vi "save_TIFF_U16array.vi"(8 "time_stamp":bool=TRUE, 9 "filename":string, 10 "Path":path=path "D:/datanew/seal/20160708_test", 11 "Image Pixels (U16)":u16[][](array[numeric])) -> ()   [LabVIEW 2014]
panel:
  out "error out":errorcluster
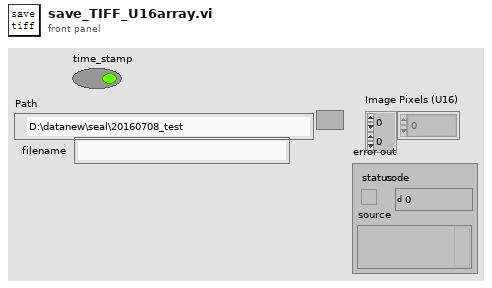
[diagram p1: front panel]
types:
  T1 = typedef "Image Type" = u32
  T2 = cluster{"Rows Per Strip":i32, "Photometric":i32, "Compression Type":i32}
  T3 = typedef "IMAQ Image.ctl" = refnum<image>
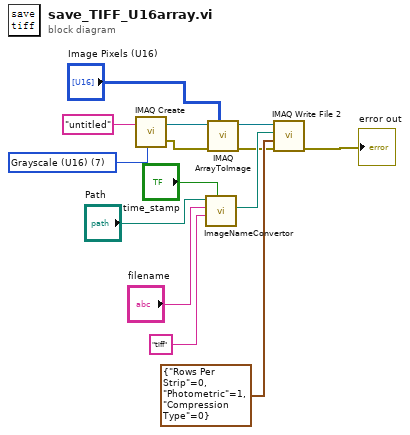
[diagram p0: block diagram]
diagram:
  w5 = T1 7 items=["Grayscale (U8)", "Grayscale (I16)", "Grayscale (SGL)", "Complex (CSG)", "RGB (U32)", "HSL (U32)", "RGB (U64)", "Grayscale (U16)"] ("Image Type")
  n1 = call "IMAQ Create"("Image Name"="untitled", "Image Type"=w5) -> ("New Image"=w7:T3, "error out"=w3:errorcluster)  [unwired: 3 in]
  n2 = call "ImageNameConvertor.vi"("time_stamp"="time_stamp", "postfix"="tiff", "filename"="filename", "Path"="Path") -> ("output"=w10:path)  [unwired: 7 in]
  n3 = call "IMAQ ArrayToImage"("Image Pixels (U16)"="Image Pixels (U16)", "error in (no error)"=w3, "Image"=w7) -> ("error out"=w2:errorcluster, "Image Out"=w9:T3)  [unwired: 7 in]
  n4 = call-poly "IMAQ Write File 2"("error in (no error)"=w2, "TIFF Options"=T2 {"Rows Per Strip"=0, "Photometric"=1, "Compression Type"=0}, "File Path"=w10, "Image"=w9) -> ("error out"=→"error out":errorcluster)  [unwired: 6 in, 1 out]
